vi "createNewDocument.vi"(8 "error in (no error)":errorcluster, 10 "Document Path":path, 11 "npoiDocument in":refnum<class "npoiDocument.lvclass">) -> (0 "error out":errorcluster, 3 "npoiDocument out":refnum<class "npoiDocument.lvclass">)   [LabVIEW 2017, in "NPOI_Document.lvlib" / "npoiDocument.lvclass"]
uses:
  npoiDocument.lvclass
  npoiDocument.lvclass/npoiDocument.ctl
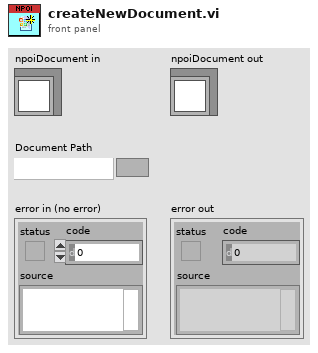
[diagram p1: front panel]
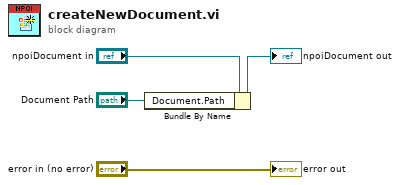
[diagram p0: block diagram]
diagram:
  n1 = Bundle By Name(cluster="npoiDocument in", "Document.Path"="Document Path") -> (→"npoiDocument out":refnum<class "npoiDocument.lvclass">)
  "error out" <- "error in (no error)"
